vi "Manhattan_distances.vi"(8 "error in":errorcluster caption="entrée d'erreur", 9 "Y":string[][](array[string]), 10 "X":string[][](array[string]), 11 "manhattan_distances":cluster{"sum_over_features":bool}={"sum_over_features"=TRUE}) -> (0 "error out":errorcluster caption="sortie d'erreur", 3 "Data":T1)   [LabVIEW 2020]
doc: "Compute the L1 distances between the vectors in X and Y.\n\nWith sum_over_features equal to False it returns the componentwise distances.\n\n\nParameters :\n\n- X : array_like\nAn array with shape (n_samples_X, n_features).\n\n- Y : array_like, optional\nAn array with shape (n_samples_Y, n_features).\n\n- sum_over_features : bool, default=True\nIf True the function returns the pairwise distance matrix else it returns the componentwise L1 pairwise-distances. Not supported for sparse matrix inputs.\n\nReturns : \n\n- D : array\nIf sum_over_features is False shape is (n_samples_X * n_samples_Y, n_features) and D contains the componentwise L1 pairwise-distances (ie. absolute difference), else shape is (n_samples_X, n_samples_Y) and D contains the pairwise L1 distances."
uses:
  Manhattan_distances.lvclass
panel:
  out "Manhattan_distances.lvclass":refnum<class "Manhattan_distances.lvclass">
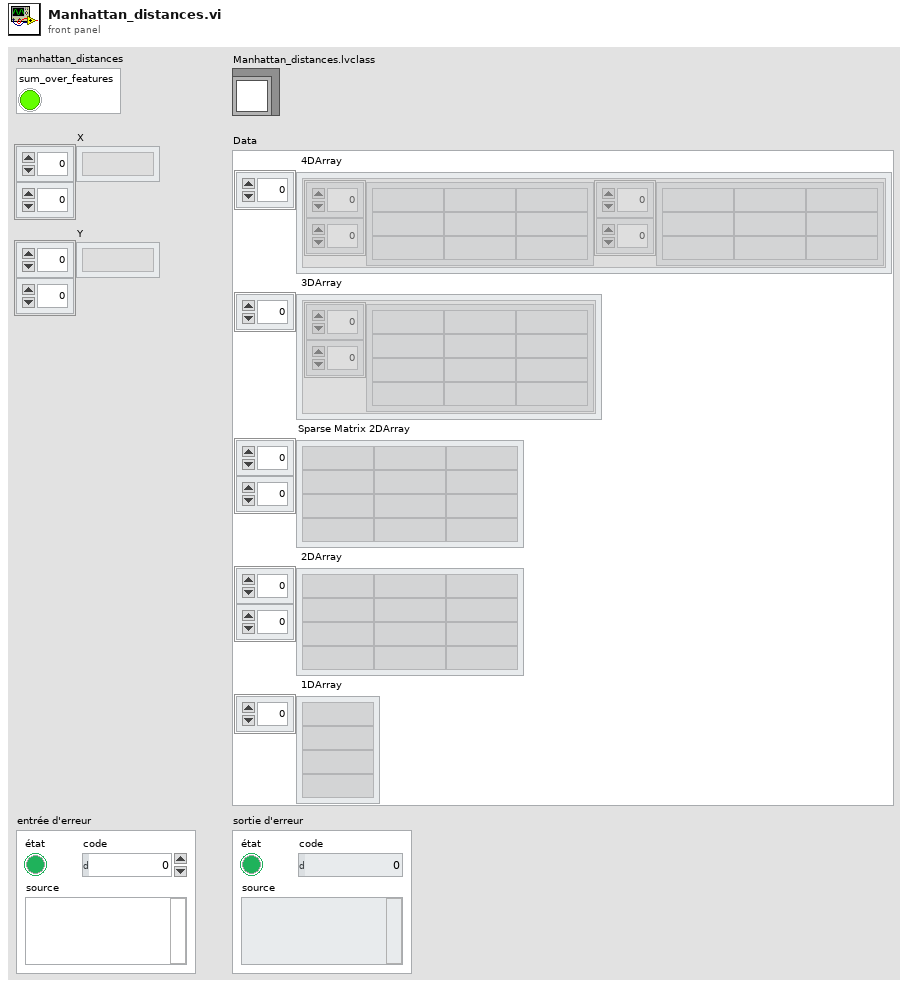
[diagram p1: front panel]
types:
  T1 = cluster{" 4DArray":cluster{"1":string[][], "2":string[][]}[], " 3DArray":cluster{"Tableau":string[][]}[], "Sparse Matrix 2DArray":string[][], " 2DArray":string[][], " 1DArray":string[]}
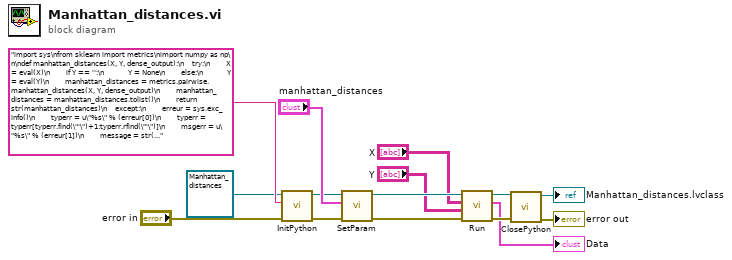
[diagram p0: block diagram]
diagram:
  n1 = call-dynamic "InitPython.vi"("error in (no error)"="error in", "Python Instruction"="import sys\nfrom sklearn import metrics\nimport numpy as np\n\ndef manhattan_distances(X, Y, dense_output):\n    try:\n        X = eval(X)\n        if Y == '':\n            Y = None\n        else:\n            Y = eval(Y)\n        manhattan_distances = metrics.pairwise.manhattan_distances(X, Y, dense_output)\n        manhattan_distances = manhattan_distances.tolist()\n        return str(manhattan_distances)\n    except:\n        erreur = sys.exc_info()\n        typerr = u\"%s\" % (erreur[0])\n        typerr = typerr[typerr.find(\"'\")+1:typerr.rfind(\"'\")]\n        msgerr = u\"%s\" % (erreur[1])\n        message = str('/!\\\\ {0} : {1}'. format(typerr,msgerr))\n        return message", "Scikit-learn en entrée"=refnum<class "Manhattan_distances.lvclass"> refnum ("Manhattan_distances.lvclass")) -> ("error out"=w9:errorcluster, "Scikit-learn en sortie"=w11:refnum<class "Manhattan_distances.lvclass">)  [unwired: 7 in]
  n2 = call-dynamic "SetParam.vi"("error in (no error)"=w9, "manhattan_distances"="manhattan_distances", "Manhattan_distances.lvclass"=w11) -> ("Manhattan_distances.lvclass"=w8:refnum<class "Manhattan_distances.lvclass">)  [unwired: 7 in, 1 out]
  n3 = call-dynamic "Run.vi"("error in (no error)"=w9, "Y"="Y", "X"="X", "Manhattan_distances.lvclass"=w8) -> ("error out"=w6:errorcluster, "Data"=→"Data":T1, "Manhattan_distances.lvclass"=w7:refnum<class "Manhattan_distances.lvclass">)  [unwired: 5 in]
  n4 = call-dynamic "ClosePython.vi"("error in (no error)"=w6, "Scikit-learn en entrée"=w7) -> ("error out"=→"error out":errorcluster, "Scikit-learn en sortie"=→"Manhattan_distances.lvclass":refnum<class "Manhattan_distances.lvclass">)  [unwired: 8 in]
